vi "Vision Processing.vi"(4 "error in (no error)":errorcluster, 6 "CameraDevRef":T1) -> ()   [LabVIEW 2011]
uses:
  <vilib>/Rock Robotics/WPI/Camera/WPI_CameraDevRef.ctl
  Robot Global Data.vi
  <vilib>/vision/NI_Vision_Development_Module.lvlib
panel:
  in  "AntiDrift":dbl
  in  "Y AbsolVal Difference":dbl=0.25
  in  "Default Shooter Speed Dump":dbl=0.4
  in  "Scale":dbl=0.85
  in  "Minimum Power":dbl=0.22
  out "Aspect Ratio":dbl[](array[numeric])
  out "Offset":dbl
  out "Raw Turret":dbl
  out "Target X Coord":dbl
  out "Target Distance":dbl
  out "Distance Array":dbl[](array[numeric])
  in  "Dead Band":dbl=0.09
  out "Number of Rectangles Visible":dbl
  out "Y Position Array":dbl[](array[numeric])
  out "X Position Array":dbl[](array[numeric])
  in  "View":bool
  out "Target Info":T2(array[cluster])
  in  "Area Size Limit":i32=444
  in  "Particle Count Limit":i32=8
  in  "Score Limits":T3={"Rect Coverage"=76.0, "Aspect Ratio"=40.0, "X Edge Strength"=40.0, "Y Edge Strength"=60.0}
  in  "Processing":enum32{"Color", "Intensity", "Intensity Open"}(tab)=enum."Intensity"
  in  "Luminance":i32=255
  in  "Saturation":i32=255
  in  "Hue":i32(knob)=65 scale=0.0..255.0
  in  "Margins":cluster{"Hue":i32, "Sat":i32, "Lum":i32}={"Hue"=20, "Sat"=27, "Lum"=30} {"Sat" scale=0.0..40.0; "Lum" scale=0.0..40.0; "Hue" scale=0.0..40.0}
  in  "Range":cluster{"Lower value":sgl, "Upper value":sgl}={"Lower value"=151.52174, "Upper value"=255.0} {"Lower value" scale=0.0..255.0; "Upper value" scale=0.0..255.0}
  in  "Range":cluster{"Lower value":sgl, "Upper value":sgl}={"Lower value"=123.804344, "Upper value"=255.0} {"Lower value" scale=0.0..255.0; "Upper value" scale=0.0..255.0}
  in  "View":bool
  out "Processed Image":T4(plugin-control)
  out "Original Image":T4(plugin-control)
  # "Instructions:\nProcessing the reflective tape that is illuminated by a ring light can be based\non color or light intensity.\nParticles within the image are scored by rectangle coverage, aspect ratio, and\nfor being hollow with a bold edge. A particle is considered a target if all scores\nare above the score limits. Particles can be annotated -- surrounded by\na rectangle and scores drawn to the left .\nTo control the number of particles being scored, use the count limit and the size\nlimit."
  # "-0.065"
  # "(in)"
  # "To debug, Enable using the View button.\nFor color processing, you can click in the image to select the color for processing."
  # "Enable by clicking the View button.\nGreen scores are above the limit, orange are below. Inner/outer rect\nindicates all passed."
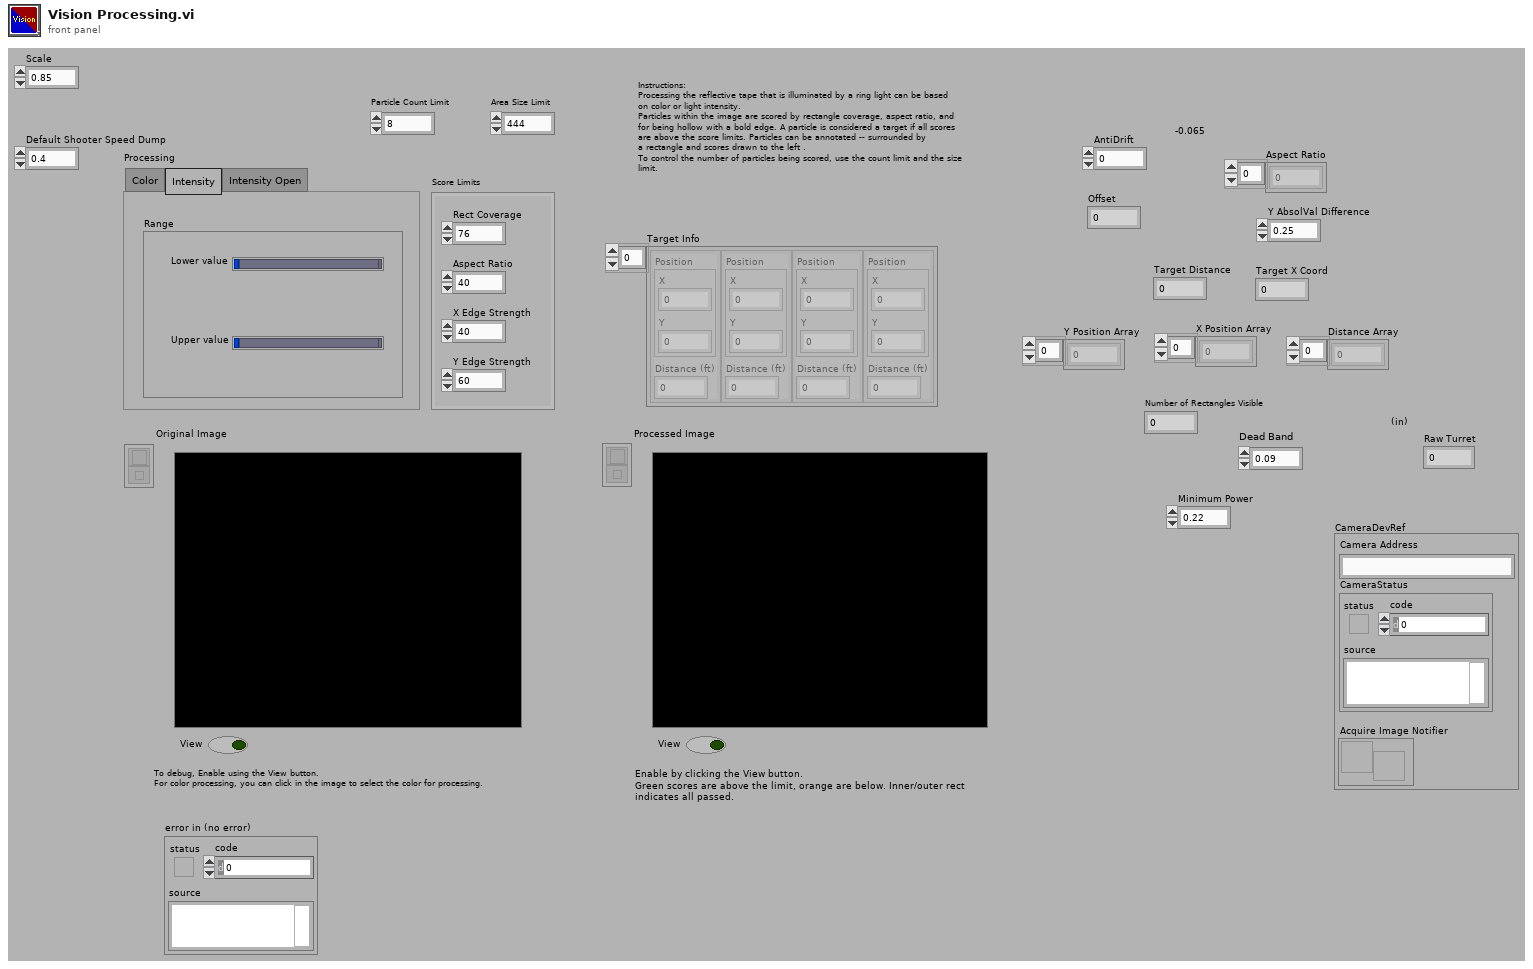
[diagram p1: front panel]
types:
  T1 = typedef "WPI_CameraDevRef.ctl" = cluster{"Camera Address":string, "CameraStatus":errorcluster, "Acquire Image Notifier":refnum<notifier>}
  T2 = cluster{"Position":cluster{"X":dbl, "Y":dbl}, "Distance (ft)":dbl}[]
  T3 = cluster{"Rect Coverage":dbl, "Aspect Ratio":dbl, "X Edge Strength":dbl, "Y Edge Strength":dbl}
  T4 = typedef "IMAQ Image.ctl" = refnum<image>
  T5 = typedef "Image Type" = u32
  T6 = enum32{"AutoM", "Close", "Dilate", "Erode", "Gradient", "Gradient out", "Gradient in", "Hit miss", "Open", "PClose", "POpen", "Thick", "Thin"}
  T7 = typedef "WPI_CameraImageSize.ctl" = enum16{"640x480", "320x240", "160x120"}
  T8 = cluster{"fps":i32, "compression":i32, "Image Size":T7}
  T9 = cluster{cluster{"Left":dbl, "Top":dbl, "Right":dbl, "Bottom":dbl}, dbl[]}[]
  T10 = cluster{"Left":dbl, "Top":dbl, "Right":dbl, "Bottom":dbl}
  T11 = cluster{"Target Center (-1 to 1)":cluster{"X":dbl, "Y":dbl}, "Distance (ft)":dbl}
  T12 = cluster{"Target Center (-1 to 1)":cluster{"X":dbl, "Y":dbl}, "Distance (ft)":dbl}[]
  T13 = typedef "WPI_JoystickDevRef.ctl" = cluster{"Device":T14}
  T14 = typedef "WPI_JoystickDeviceEnum.ctl" = enum16{"USB 1", "USB 2", "USB 3", "USB 4", "Kinect 1", "Kinect 2"}
  T15 = typedef "WPI_JoystickButtonState.ctl" = cluster{"Button 1":bool, "Button 2":bool, "Button 3":bool, "Button 4":bool, "Button 5":bool, "Button 6":bool, "Button 7":bool, "Button 8":bool, "Button 9":bool, "Button 10":bool, "Button 11":bool, "Button 12":bool}
  T16 = cluster{"axis 1 (x)":dbl, "axis 2 (y)":dbl, "axis 3 (throttle)":dbl, "axis 4":dbl, "axis 5":dbl, "axis 6":dbl}
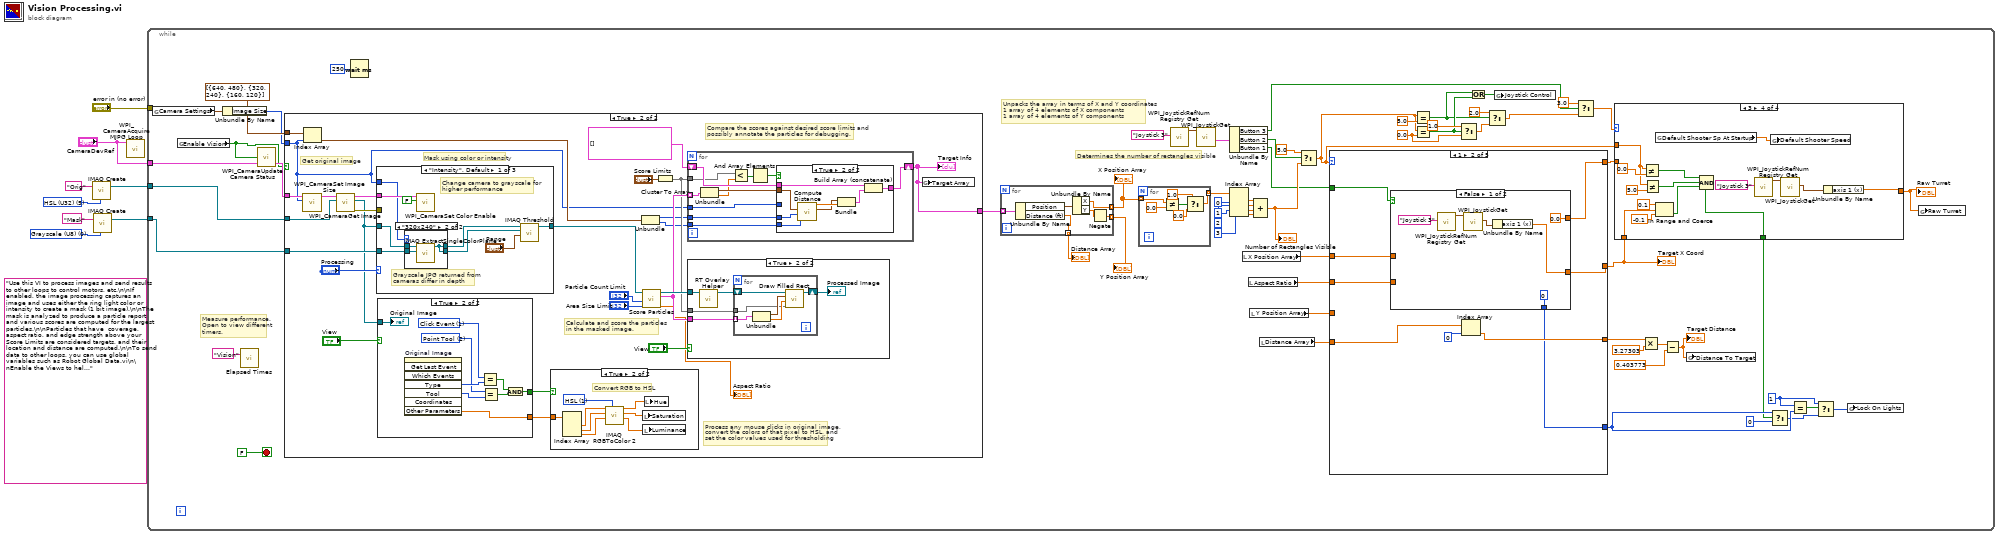
[diagram p0: block diagram]
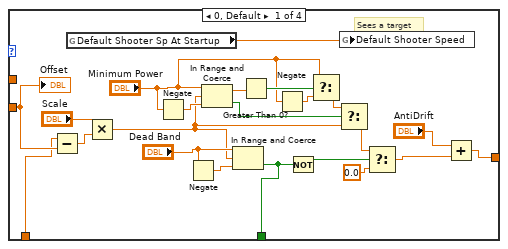
[diagram p2: hidden frame]
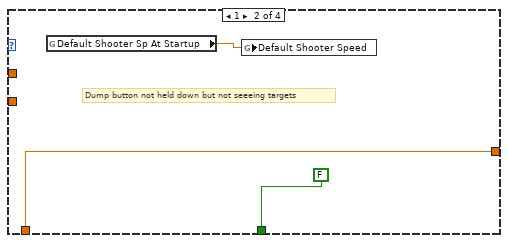
[diagram p3: hidden frame]
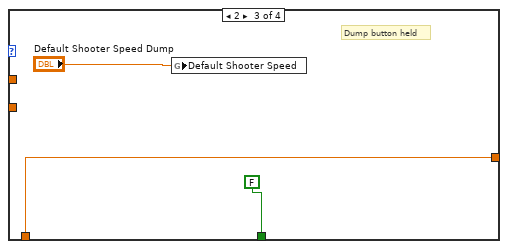
[diagram p4: hidden frame]
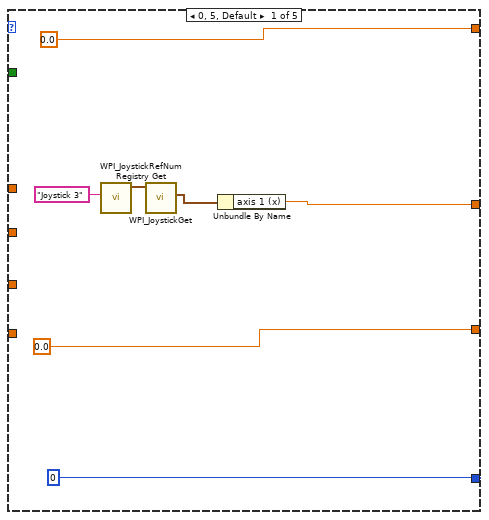
[diagram p5: hidden frame]
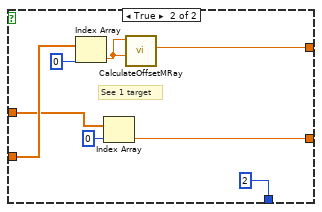
[diagram p6: hidden frame]
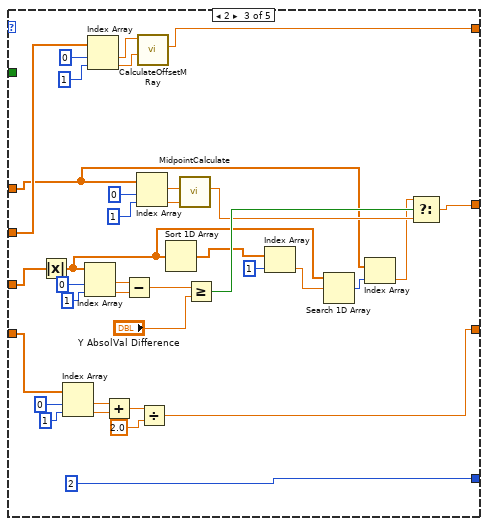
[diagram p7: hidden frame]
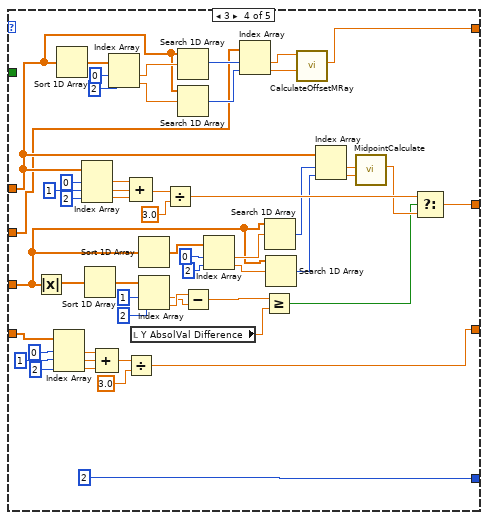
[diagram p8: hidden frame]
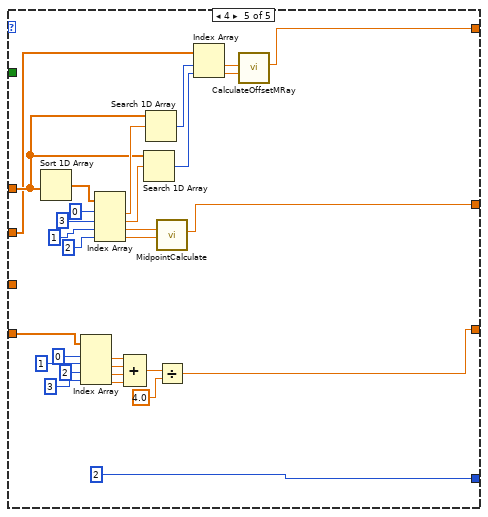
[diagram p9: hidden frame]
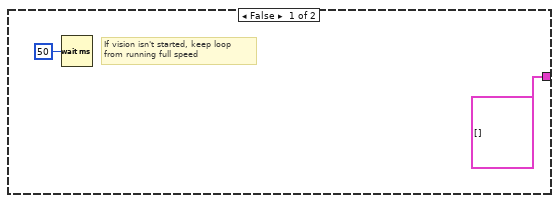
[diagram p10: hidden frame]
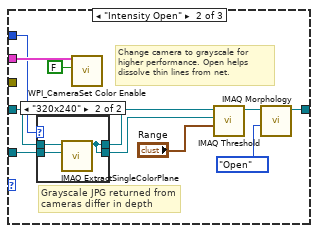
[diagram p13: hidden frame]
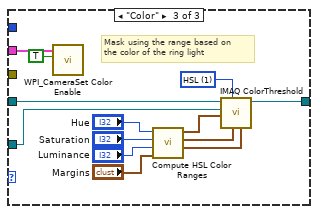
[diagram p15: hidden frame]
diagram:
  w3 = T5 0 items=["Grayscale (U8)", "Grayscale (I16)", "Grayscale (SGL)", "Complex (CSG)", "RGB (U32)", "HSL (U32)", "RGB (U64)", "Grayscale (U16)"] ("Image Type")
  (unwired) "Use this VI to process images and send results to other loops to control motors, etc.\n\nIf enabled, the image processing captures an image and uses either the ring light color or intensity to create a mask (1 bit image).\n\nThe mask is analyzed to produce a particle report and various scores are computed for the largest particles.\n\nParticles that have  coverage, aspect ratio, and edge strength above your Score Limits are considered targets, and their location and distance are computed.\n\nTo send data to other loops, you can use global variables such as Robot Global Data.vi\n\nEnable the Views to help debug color settings. Disable the View to speed up processing."
  w7 = T5 5 items=["Grayscale (U8)", "Grayscale (I16)", "Grayscale (SGL)", "Complex (CSG)", "RGB (U32)", "HSL (U32)", "RGB (U64)", "Grayscale (U16)"] ("Image Type")
  n1 = call "IMAQ Create"("Image Name"="Orig", "Image Type"=w7) -> ("New Image"=w6:T4)  [unwired: 2 in, 2 out]
  n2 = call "IMAQ Create"("Image Name"="Mask", "Image Type"=w3) -> ("New Image"=w1:T4)  [unwired: 2 in, 2 out]
  n3 = call <vilib>:"WPI_CameraAcquire MJPG Loop.vi"("CameraDevRef"="CameraDevRef") -> ()  [unwired: 11 in]
  n4 = while {
    tunnel: w6 -> [w70]
    tunnel: "CameraDevRef" -> [w69]
    tunnel: "error in (no error)" -> [_]
    tunnel: w1 -> [w65]
    stop <- FALSE stop-if-true
    w18 = 0.0 ("y")
    w35 = 1 ("y")
    # "Determines the number of rectangles visible"
    # "Unpacks the array in terms of X and Y coordinates\n1 array of 4 elements of X components\n1 array of 4 elements of Y components"
    # "Measure performance.\nOpen to view different\ntimers."
    n5 = global read "Robot Global Data.vi" "Camera Settings"() -> (w63:T8)
    n6 = global read "Robot Global Data.vi" "Enable Vision"() -> (w67:bool)
    n7 = Unbundle By Name(w63) -> ("Image Size"=w62:T7)
    n8 = call "Elapsed Times.vi"("Call Name"="Vision") -> ()  [unwired: 2 in, 1 out]
    n9 = call <vilib>:"WPI_CameraUpdate Camera Status.vi"("CameraDevRef In"=w69, "Enable Vision"=w67) -> ("CameraDevRef Out"=w68:T1)  [unwired: 3 in]
    n10 = case shown="True" w67 {
      tunnel: w70 -> [_ w295]
      tunnel: w68 -> [_ w291]
      tunnel: w65 -> [_ w282]
      tunnel: cluster{i32, i32}[] [{640, 480}, {320, 240}, {160, 120}] -> [_ w286]
      tunnel: w62 -> [_ w279]
      tunnel: [T2 [] w280] -> w61
      frame False {
        # "If vision isn't started, keep loop\nfrom running full speed"
        n11 = Wait (ms)(milliseconds to wait=u32 50) -> ()  [unwired: 1 out]
      }
      frame True {
        # "Compare the scores against desired score limits and\npossibly annotate the particles for debugging."
        # "Process any mouse clicks in original image,\nconvert the colors of that pixel to HSL, and\nset the color values used for thresholding"
        # "Calculate and score the particles\nin the masked image."
        # "Mask using color or intensity"
        # "Get original image"
        n12 = call <vilib>:"WPI_CameraSet Image Size.vi"("Image Size"=w279, "CameraDevRef"=w291) -> ("CameraDevRef Out"=w292:T1)  [unwired: 8 in, 1 out]
        n13 = Index Array(array=w286, index=w279) -> (element=w283:cluster{i32, i32})
        n14 = call <vilib>:"WPI_CameraGet Image.vi"("Image"=w295, "CameraDevRef"=w292) -> ("error out"=w293:errorcluster, "Image Out"=w281:T4, "CameraDevRef Out"=w294:T1)  [unwired: 7 in]
        n15 = case shown="\"Intensity\", Default" "Processing" {
          tunnel: w281 -> [w317 w329 w355]
          tunnel: [w320 w334 w354] -> w289
          tunnel: w294 -> [w318 w332 w345]
          tunnel: w293 -> [_ _ _]
          tunnel: w282 -> [w316 w330 w343]
          tunnel: w279 -> [w315 w331 _]
          frame "Intensity", Default {
            # "Grayscale JPG returned from\ncameras differ in depth"
            # "Change camera to grayscale for\nhigher performance"
            n16 = case shown="\"320x240\"" w315 {
              tunnel: w317 -> [w323 w326]
              tunnel: w316 -> [w322 w325]
              tunnel: [w323 w324] -> w314
              tunnel: [w322 w324] -> w313
              frame "640x480", Default {
              }
              frame "320x240" {
                n17 = call "IMAQ ExtractSingleColorPlane"("Image Dst"=w325, "Image Src"=w326) -> ("Image Dst Out"=w324:T4)  [unwired: 8 in, 1 out]
              }
            }
            n18 = call <vilib>:"WPI_CameraSet Color Enable.vi"("Color Enabled"=FALSE, "CameraDevRef"=w318) -> ()  [unwired: 8 in, 2 out]
            n19 = call "IMAQ Threshold"("Range"="Range", "Image Dst"=w313, "Image Src"=w314) -> ("Image Dst Out"=w320:T4)  [unwired: 3 in, 5 out]
          }
          frame "Intensity Open" {
            # "Grayscale JPG returned from\ncameras differ in depth"
            # "Change camera to grayscale for\nhigher performance. Open helps\ndissolve thin lines from net."
            n20 = case shown="\"320x240\"" w331 {
              tunnel: w329 -> [w339 w342]
              tunnel: w330 -> [w338 w341]
              tunnel: [w339 w340] -> w328
              tunnel: [w338 w340] -> w327
              frame "640x480", Default {
              }
              frame "320x240" {
                n21 = call "IMAQ ExtractSingleColorPlane"("Image Dst"=w341, "Image Src"=w342) -> ("Image Dst Out"=w340:T4)  [unwired: 8 in, 1 out]
              }
            }
            n22 = call <vilib>:"WPI_CameraSet Color Enable.vi"("Color Enabled"=FALSE, "CameraDevRef"=w332) -> ()  [unwired: 8 in, 2 out]
            n23 = call "IMAQ Threshold"("Range"="Range", "Image Dst"=w327, "Image Src"=w328) -> ("Image Dst Out"=w335:T4)  [unwired: 3 in, 5 out]
            n24 = call "IMAQ Morphology"("Operation"=T6."Open", "Image Src"=w335) -> ("Image Dst Out"=w334:T4)  [unwired: 8 in, 1 out]
          }
          frame "Color" {
            w353 = u16 1 items=["RGB", "HSL", "HSV", "HSI"] ("Color Mode")
            # "Mask using the range based on\nthe color of the ring light"
            n25 = call <vilib>:"WPI_CameraSet Color Enable.vi"("Color Enabled"=TRUE, "CameraDevRef"=w345) -> ()  [unwired: 8 in, 2 out]
            n26 = call "Compute HSL Color Ranges.vi"("Margins"="Margins", "Luminance"="Luminance", "Saturation"="Saturation", "Hue"="Hue") -> ("Lum Range"=w350:cluster{i32, i32}, "Sat Range"=w351:cluster{i32, i32}, "Hue Range"=w352:cluster{i32, i32})  [unwired: 5 in]
            n27 = call "IMAQ ColorThreshold"("Blue or Luma or Val or Inten Range"=w350, "Green or Sat Range"=w351, "Color Mode"=w353, "Red or Hue Range"=w352, "Image Dst"=w343, "Image Src"=w355) -> ("Image Dst Out"=w354:T4)  [unwired: 4 in, 1 out]
          }
        }
        n28 = case shown="True" "View" {
          tunnel: w281 -> [_ w375]
          tunnel: [_ w370] -> w288
          tunnel: [_ w367] -> w287
          frame False {
          }
          frame True {
            w368 = 2 items=["None", "Selection Tool", "Point Tool", "Line Tool", "Rectangle Tool", "Oval Tool", "Polygon Tool", "ClosedFreehandTool", "Annulus Tool", "Rotated Rectangle Tool", "Zoom Tool", "Pan Tool", "Polyline Tool", "Freehand Tool"] ("Tool")
            w369 = 1 items=["No Event"=0, "Click Event"=1, "Draw Event"=2, "Size Event"=4, "Scroll Event"=5, "Double Click Event"=8] ("Type")
            n29 = invoke on="Original Image" class="ImageControl" method="Get Last Event"() -> ("Type"=w371:i32, "Tool"=w374:i32, "Other Parameters"=w367:sgl[])  [unwired: 8 in, 5 out]
            n30 = Equal?(x=w369, y=w371) -> (x = y?=w372:bool)
            n31 = Equal?(x=w368, y=w374) -> (x = y?=w373:bool)
            n32 = And(x=w372, y=w373) -> (x .and. y?=w370:bool)
            "Original Image" <- w375
          }
        }
        n33 = case shown="True" w288 {
          tunnel: w287 -> [_ w312]
          frame False {
          }
          frame True {
            w311 = u16 1 items=["RGB", "HSL", "HSV", "HSI", "CIE L*a*b*", "CIE XYZ"] ("Color Mode")
            # "Convert RGB to HSL"
            n34 = Index Array(array=w312) -> (element #1=w310:sgl, element #2=w308:sgl, element #3=w306:sgl)  [unwired: 3 in]
            n35 = call "IMAQ RGBToColor 2"("Color Mode"=w311, "Blue value"=w306, "Green value"=w308, "Red value"=w310) -> ("Blue or Luma or Val or Inten or Z or b*value"=w305:dbl, "Green or Sat or Y or a* value"=w307:dbl, "Red or Hue or X or L* value"=w309:dbl)  [unwired: 4 in, 1 out]
            n36 = local write "Saturation"(w307) -> ()
            n37 = local write "Luminance"(w305) -> ()
            n38 = local write "Hue"(w309) -> ()
          }
        }
        n39 = Unbundle(w283) -> (w285:i32, w284:i32)
        n40 = call "Score Particles.vi"("Area Size Limit"="Area Size Limit", "Particle Count Limit"="Particle Count Limit", "Image Refnum in"=w289) -> ("Aspect Ratio"=→"Aspect Ratio":dbl[], "Scored Particle Info"=w300:T9, "Image Refnum out"=w303:T4)  [unwired: 6 in]
        n41 = Cluster To Array(cluster="Score Limits") -> (array=w298:dbl[])
        n42 = for {
          shift-right: [w385] -> w280
          shift-left: T2 [] -> [w386]
          tunnel: w285 -> [w384]
          tunnel: w300 -> [w382] mode=indexing
          tunnel: w298 -> [w377]
          tunnel: w279 -> [w381]
          tunnel: w284 -> [w376]
          n43 = Unbundle(w382) -> (w383:T10, w378:dbl[])
          n44 = Less?(x=w377, y=w378) -> (x < y?=w380:bool[])
          n45 = And Array Elements(Boolean array=w380) -> (logical AND=w379:bool)
          n46 = case shown="True" w379 {
            tunnel: w386 -> [w387 w395]
            tunnel: [w387 w394] -> w385
            tunnel: w383 -> [_ w390]
            tunnel: w384 -> [_ w392]
            tunnel: w381 -> [_ _]
            tunnel: w376 -> [_ w389]
            frame False {
            }
            frame True {
              n47 = call "Compute Distance.vi"("Y Image Resolution"=w389, "X Image Resolution"=w392, "Bounding Box"=w390) -> ("Target Center (-1 to 1)"=w388:cluster{"X":dbl, "Y":dbl}, "Distance (ft)"=w391:dbl)  [unwired: 7 in]
              n48 = Bundle("Target Center (-1 to 1)"=w388, "Distance (ft)"=w391) -> (w393:T11)  [unwired: 1 in]
              n49 = Build Array (concatenate)(w395, w393) -> (w394:T12)
            }
          }
        }
        "Target Info" <- w280
        n50 = case shown="True" "View" {
          tunnel: w303 -> [_ w357]
          tunnel: w300 -> [_ w359]
          tunnel: w298 -> [_ w358]
          frame False {
          }
          frame True {
            n51 = call "RT Overlay Helper.vi"("Refnum in"=w357) -> ("Refnum out"=w360:T4)  [unwired: 10 in]
            n52 = for {
              shift-right: [w365] -> w356
              shift-left: w360 -> [w366]
              tunnel: w359 -> [w362] mode=indexing
              tunnel: w358 -> [w361]
              n53 = Unbundle(w362) -> (w363:T10, w364:dbl[])
              n54 = call "Draw Filled Rect.vi"("Limits"=w361, "Scores"=w364, "Bounding Box"=w363, "image in"=w366) -> ("image out"=w365:T4)  [unwired: 7 in]
            }
            "Processed Image" <- w356
          }
        }
        n55 = global write "Robot Global Data.vi" "Target Array"(w280) -> ()
      }
    }
    n56 = Wait (ms)(milliseconds to wait=u32 250) -> ()  [unwired: 1 out]
    n57 = for {
      tunnel: [w273] -> w41 mode=indexing
      tunnel: [w274] -> w51 mode=indexing
      tunnel: w61 -> [w271] mode=indexing
      tunnel: [w270] -> w53 mode=indexing
      n58 = Unbundle By Name(w271) -> ("Position"=w275:cluster{"X":dbl, "Y":dbl}, "Distance (ft)"=w270:dbl)
      n59 = Unbundle By Name(w275) -> ("X"=w274:dbl, "Y"=w272:dbl)
      n60 = Negate(x=w272) -> (-x=w273:dbl)
    }
    "X Position Array" <- w51
    "Y Position Array" <- w41
    "Distance Array" <- w53
    n61 = for {
      tunnel: w51 -> [w119] mode=indexing
      tunnel: [w115] -> w50 mode=indexing
      n62 = Not Equal?(x=w119, y=0.0) -> (x != y?=w118:bool)
      n63 = Select(t=1.0, s=w118, f=0.0) -> (s? t:f=w115:dbl)
    }
    n64 = call <vilib>:"WPI_JoystickRefNum Registry Get.vi"("refnum name"="Joystick 3") -> ("JoystickDevRef"=w40:T13)  [unwired: 9 in, 1 out]
    n65 = call <vilib>:"WPI_JoystickGet.vi"("JoystickDevRef"=w40) -> ("Buttons"=w38:T15)  [unwired: 4 in, 2 out]
    n66 = Unbundle By Name(w38) -> ("Button 3"=w12:bool, "Button 2"=w37:bool, "Button 1"=w9:bool)
    n67 = Index Array(array=w50, index #1=0 ("index"), index #2=1 ("index"), index #3=2 ("index"), index #4=3 ("index")) -> (element #1=w48:dbl, element #2=w49:dbl, element #3=w47:dbl, element #4=w46:dbl)
    n68 = local read "X Position Array"() -> (w52:dbl[])
    n69 = local read "Aspect Ratio"() -> (w30:dbl[])
    n70 = local read "Y Position Array"() -> (w54:dbl[])
    n71 = Compound Arithmetic op=ADD(w48, w49, w47, w46) -> (w31:dbl)
    "Number of Rectangles Visible" <- w31
    n72 = local read "Distance Array"() -> (w55:dbl[])
    n73 = Select(t=5.0, s=w37, f=w31) -> (s? t:f=w10:dbl)
    n74 = case shown="1" w10 {
      tunnel: w52 -> [_ w134 w152 w194 w245]
      tunnel: [w123 w133 w176 w228 w268] -> w28
      tunnel: w54 -> [_ _ w175 w206 _]
      tunnel: w55 -> [_ w130 w164 w237 w265]
      tunnel: [0 w128 2 2 2] -> w34
      tunnel: [0.0 ("Offset") w135 w181 w187 w254] -> w29
      tunnel: w30 -> [_ w136 w184 w190 w240]
      tunnel: [0.0 w129 w159 w230 w255] -> w23
      tunnel: w9 -> [_ w132 _ _ _]
      frame 0, 5, Default {
        n75 = call <vilib>:"WPI_JoystickRefNum Registry Get.vi"("refnum name"="Joystick 3") -> ("JoystickDevRef"=w122:T13)  [unwired: 9 in, 1 out]
        n76 = call <vilib>:"WPI_JoystickGet.vi"("JoystickDevRef"=w122) -> ("Axes"=w124:T16)  [unwired: 4 in, 2 out]
        n77 = Unbundle By Name(w124) -> ("axis 1 (x)"=w123:dbl)
      }
      frame 1 {
        n78 = case shown="False" w132 {
          tunnel: w136 -> [_ w150]
          tunnel: [0.0 ("Offset") w147] -> w135
          tunnel: w134 -> [_ w145]
          tunnel: [w139 w144] -> w133
          tunnel: [0 2] -> w128
          frame False {
            n79 = call <vilib>:"WPI_JoystickRefNum Registry Get.vi"("refnum name"="Joystick 3") -> ("JoystickDevRef"=w140:T13)  [unwired: 9 in, 1 out]
            n80 = call <vilib>:"WPI_JoystickGet.vi"("JoystickDevRef"=w140) -> ("Axes"=w141:T16)  [unwired: 4 in, 2 out]
            n81 = Unbundle By Name(w141) -> ("axis 1 (x)"=w139:dbl)
          }
          frame True {
            # "See 1 target"
            n82 = Index Array(array=w150, index=0) -> (element=w148:dbl)
            n83 = Index Array(array=w145, index=0) -> (element=w144:dbl)
            n84 = call "CalculateOffsetMRay.vi"("AR2"=w148, "AR1"=w148) -> ("Offset"=w147:dbl)  [unwired: 9 in]
          }
        }
        n85 = Index Array(array=w130, index=0) -> (element=w129:dbl)
      }
      frame 2 {
        n86 = Absolute Value(x=w175) -> (abs(x)=w155:dbl[])
        n87 = Index Array(array=w164, index #1=0 ("index"), index #2=1 ("index")) -> (element #1=w162:dbl, element #2=w163:dbl)
        n88 = Index Array(array=w155, index #1=0 ("index"), index #2=1 ("index")) -> (element #1=w171:dbl, element #2=w172:dbl)
        n89 = Index Array(array=w184, index #1=0 ("index"), index #2=1 ("index")) -> (element #1=w183:dbl, element #2=w182:dbl)
        n90 = Add(x=w162, y=w163) -> (x+y=w161:dbl)
        n91 = Subtract(x=w171, y=w172) -> (x-y=w170:dbl)
        n92 = Index Array(array=w152, index #1=0 ("index"), index #2=1 ("index")) -> (element #1=w177:dbl, element #2=w178:dbl)
        n93 = call "CalculateOffsetMRay.vi"("AR2"=w182, "AR1"=w183) -> ("Offset"=w181:dbl)  [unwired: 9 in]
        n94 = Divide(x=w161, y=2.0) -> (x/y=w159:dbl)
        n95 = Sort 1D Array(array=w155) -> (sorted array=w157:dbl[])
        n96 = call "MidpointCalculate.vi"("X2"=w178, "X1"=w177) -> ("Midpoint"=w167:dbl)  [unwired: 9 in]
        n97 = Greater Or Equal?(x=w170, y="Y AbsolVal Difference") -> (x >= y?=w168:bool)
        n98 = Index Array(array=w157, index=1) -> (element=w154:dbl)
        n99 = Search 1D Array(1D array=w155, element=w154) -> (index of element=w153:i32)  [unwired: 1 in]
        n100 = Index Array(array=w152, index=w153) -> (element=w151:dbl)
        n101 = Select(t=w151, s=w168, f=w167) -> (s? t:f=w176:dbl)
      }
      frame 3 {
        n102 = Absolute Value(x=w206) -> (abs(x)=w227:dbl[])
        n103 = Index Array(array=w237, index #1=0 ("index"), index #2=1 ("index"), index #3=2 ("index")) -> (element #1=w233:dbl, element #2=w234:dbl, element #3=w235:dbl)
        n104 = Sort 1D Array(array=w194) -> (sorted array=w198:dbl[])
        n105 = Index Array(array=w194, index #1=0 ("index"), index #2=1 ("index"), index #3=2 ("index")) -> (element #1=w215:dbl, element #2=w217:dbl, element #3=w216:dbl)
        n106 = Sort 1D Array(array=w227) -> (sorted array=w211:dbl[])
        n107 = Compound Arithmetic op=ADD(w233, w234, w235) -> (w232:dbl)
        n108 = Index Array(array=w198, index #1=0 ("index"), index #2=2 ("index")) -> (element #1=w195:dbl, element #2=w193:dbl)
        n109 = Divide(x=w232, y=3.0) -> (x/y=w230:dbl)
        n110 = Compound Arithmetic op=ADD(w215, w217, w216) -> (w214:dbl)
        n111 = local read "Y AbsolVal Difference"() -> (w221:dbl)
        n112 = Sort 1D Array(array=w206) -> (sorted array=w210:dbl[])
        n113 = Index Array(array=w211, index #1=1 ("index"), index #2=2 ("index")) -> (element #1=w223:dbl, element #2=w224:dbl)
        n114 = Divide(x=w214, y=3.0) -> (x/y=w212:dbl)
        n115 = Search 1D Array(1D array=w194, element=w195) -> (index of element=w192:i32)  [unwired: 1 in]
        n116 = Search 1D Array(1D array=w194, element=w193) -> (index of element=w191:i32)  [unwired: 1 in]
        n117 = Subtract(x=w224, y=w223) -> (x-y=w222:dbl)
        n118 = Index Array(array=w210, index #1=0 ("index"), index #2=2 ("index")) -> (element #1=w207:dbl, element #2=w205:dbl)
        n119 = Index Array(array=w190, index #1=w192, index #2=w191) -> (element #1=w189:dbl, element #2=w188:dbl)
        n120 = Greater Or Equal?(x=w222, y=w221) -> (x >= y?=w199:bool)
        n121 = Search 1D Array(1D array=w206, element=w207) -> (index of element=w204:i32)  [unwired: 1 in]
        n122 = Search 1D Array(1D array=w206, element=w205) -> (index of element=w203:i32)  [unwired: 1 in]
        n123 = call "CalculateOffsetMRay.vi"("AR2"=w188, "AR1"=w189) -> ("Offset"=w187:dbl)  [unwired: 9 in]
        n124 = Index Array(array=w194, index #1=w204, index #2=w203) -> (element #1=w201:dbl, element #2=w202:dbl)
        n125 = call "MidpointCalculate.vi"("X2"=w202, "X1"=w201) -> ("Midpoint"=w200:dbl)  [unwired: 9 in]
        n126 = Select(t=w212, s=w199, f=w200) -> (s? t:f=w228:dbl)
      }
      frame 4 {
        n127 = Sort 1D Array(array=w245) -> (sorted array=w269:dbl[])
        n128 = Index Array(array=w265, index #1=0 ("index"), index #2=1 ("index"), index #3=2 ("index"), index #4=3 ("index")) -> (element #1=w262:dbl, element #2=w261:dbl, element #3=w260:dbl, element #4=w259:dbl)
        n129 = Index Array(array=w269, index #1=0 ("index"), index #2=3 ("index"), index #3=1 ("index"), index #4=2 ("index")) -> (element #1=w246:dbl, element #2=w247:dbl, element #3=w253:dbl, element #4=w252:dbl)
        n130 = Compound Arithmetic op=ADD(w262, w261, w260, w259) -> (w258:dbl)
        n131 = Search 1D Array(1D array=w245, element=w247) -> (index of element=w242:i32)  [unwired: 1 in]
        n132 = Search 1D Array(1D array=w245, element=w246) -> (index of element=w241:i32)  [unwired: 1 in]
        n133 = call "MidpointCalculate.vi"("X2"=w252, "X1"=w253) -> ("Midpoint"=w268:dbl)  [unwired: 9 in]
        n134 = Divide(x=w258, y=4.0) -> (x/y=w255:dbl)
        n135 = Index Array(array=w240, index #1=w241, index #2=w242) -> (element #1=w244:dbl, element #2=w243:dbl)
        n136 = call "CalculateOffsetMRay.vi"("AR2"=w243, "AR1"=w244) -> ("Offset"=w254:dbl)  [unwired: 9 in]
      }
    }
    "Target X Coord" <- w28
    n137 = Equal?(x=w10, y=5.0) -> (x = y?=w16:bool)
    n138 = Equal?(x=w10, y=w18) -> (x = y?=w17:bool)
    n139 = Select(t=1.0, s=w17, f=w18) -> (s? t:f=w21:dbl)
    n140 = Or(x=w16, y=w17) -> (x .or. y?=w15:bool)
    n141 = Select(t=2.0, s=w16, f=w21) -> (s? t:f=w14:dbl)
    n142 = global write "Robot Global Data.vi" "Joystick Control"(w15) -> ()
    n143 = Select(t=3.0, s=w12, f=w14) -> (s? t:f=w13:dbl)
    n144 = case shown="3" w13 {
      tunnel: w29 -> [w92 _ _ _]
      tunnel: w28 -> [w91 w96 w99 w103]
      tunnel: [w74 w96 w99 w110] -> w59
      tunnel: [w77 FALSE FALSE w105] -> w27
      tunnel: w10 -> [_ _ _ w104]
      frame 0, Default {
        # "Sees a target"
        n145 = Subtract(x=w91, y=w92) -> (x-y=w89:dbl)
        n146 = global read "Robot Global Data.vi" "Default Shooter Sp At Startup"() -> (w72:dbl)
        n147 = Multiply(x="Scale", y=w89) -> (x*y=w80:dbl)
        n148 = Negate(x="Minimum Power") -> (-x=w87:dbl)
        n149 = Negate(x="Dead Band") -> (-x=w93:dbl)
        n150 = In Range and Coerce(upper limit="Minimum Power", x=w80, lower limit=w87) -> (coerced(x)=w83:dbl, In Range?=w84:bool)
        n151 = In Range and Coerce(upper limit="Dead Band", x=w80, lower limit=w93) -> (In Range?=w77:bool)  [unwired: 1 out]
        n152 = Greater Than 0?(x=w83) -> (x > 0?=w82:bool)
        n153 = Negate(x="Minimum Power") -> (-x=w79:dbl)
        n154 = Not(x=w77) -> (.not. x?=w78:bool)
        n155 = Select(t="Minimum Power", s=w82, f=w79) -> (s? t:f=w81:dbl)
        n156 = Select(t=w81, s=w84, f=w80) -> (s? t:f=w85:dbl)
        n157 = global write "Robot Global Data.vi" "Default Shooter Speed"(w72) -> ()
        n158 = Select(t=w85, s=w78, f=0.0) -> (s? t:f=w75:dbl)
        n159 = Add(x="AntiDrift", y=w75) -> (x+y=w74:dbl)
        "Offset" <- w92
      }
      frame 1 {
        # "Dump button not held down but not seeeing targets"
        n160 = global read "Robot Global Data.vi" "Default Shooter Sp At Startup"() -> (w94:dbl)
        n161 = global write "Robot Global Data.vi" "Default Shooter Speed"(w94) -> ()
      }
      frame 2 {
        # "Dump button held"
        n162 = global write "Robot Global Data.vi" "Default Shooter Speed"("Default Shooter Speed Dump") -> ()
      }
      frame 3 {
        n163 = Not Equal?(x=w104, y=0.0) -> (x != y?=w106:bool)
        n164 = Not Equal?(x=w104, y=5.0) -> (x != y?=w107:bool)
        n165 = In Range and Coerce(upper limit=0.1, x=w103, lower limit=-0.1) -> (In Range?=w101:bool)  [unwired: 1 out]
        n166 = global read "Robot Global Data.vi" "Default Shooter Sp At Startup"() -> (w114:dbl)
        n167 = Compound Arithmetic op=AND(w106, w107, w101) -> (w105:bool)
        n168 = call <vilib>:"WPI_JoystickRefNum Registry Get.vi"("refnum name"="Joystick 3") -> ("JoystickDevRef"=w113:T13)  [unwired: 9 in, 1 out]
        n169 = global write "Robot Global Data.vi" "Default Shooter Speed"(w114) -> ()
        n170 = call <vilib>:"WPI_JoystickGet.vi"("JoystickDevRef"=w113) -> ("Axes"=w112:T16)  [unwired: 4 in, 2 out]
        n171 = Unbundle By Name(w112) -> ("axis 1 (x)"=w110:dbl)
      }
    }
    "Raw Turret" <- w59
    n172 = Multiply(x=w23, y=3.27303) -> (x*y=w26:dbl)
    n173 = Subtract(x=w26, y=0.403773) -> (x-y=w57:dbl)
    "Target Distance" <- w57
    n174 = global write "Robot Global Data.vi" "Distance To Target"(w57) -> ()
    n175 = Select(t=w34, s=w27, f=0) -> (s? t:f=w32:i32)
    n176 = Equal?(x=w35, y=w34) -> (x = y?=w36:bool)
    n177 = Select(t=w35, s=w36, f=w32) -> (s? t:f=w58:i32)
    n178 = global write "Robot Global Data.vi" "Lock On Lights"(w58) -> ()
    n179 = global write "Robot Global Data.vi" "Raw Turret"(w59) -> ()
  }
